vi "Translate Core.vi"(8 "error in (no error)":errorcluster, 10 "Translation":T1, 11 "Selection in":refnum<class "Selection.lvclass">) -> (0 "error out":errorcluster, 3 "Selection out":refnum<class "Selection.lvclass">)   [LabVIEW 2017, in "LV Image Editor Framework.lvlib" / "Selection.lvclass"]
uses:
  <vilib>/LIEF/Forms/Selection/Selection.lvclass
  <vilib>/Utility/miscctls.llb/LVPoint32TypeDef.ctl
  <vilib>/LIEF/Forms/Shape/Shape.lvclass
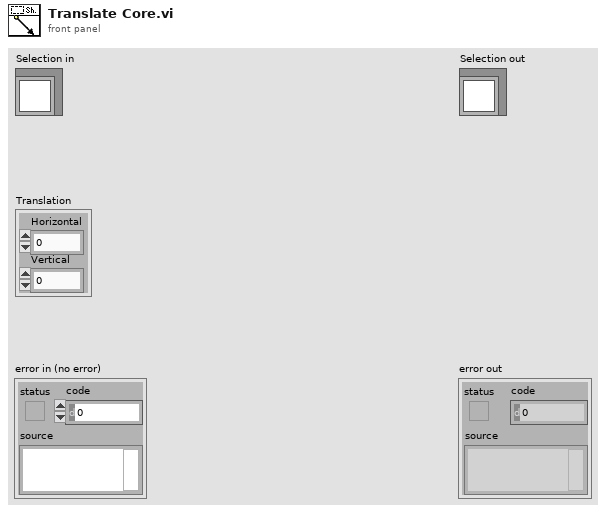
[diagram p1: front panel]
types:
  T1 = typedef "LVPoint32TypeDef.ctl" = cluster{"Horizontal":i32, "Vertical":i32}
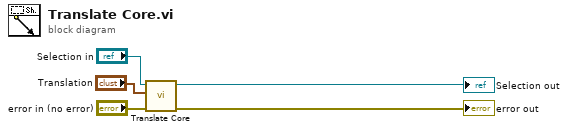
[diagram p0: block diagram]
diagram:
  n1 = call-parent "Translate Core.vi"("error in (no error)"="error in (no error)", "Translation"="Translation", "Shape in"="Selection in") -> ("error out"=→"error out":errorcluster, "Shape out"=→"Selection out":refnum<class "Selection.lvclass">)  [unwired: 7 in]
